vi "Read Credentials.vi"(8 "error in (no error)":errorcluster, 11 "AWS Core in":refnum<class "Session.lvclass">) -> (0 "error out":errorcluster, 2 "Credentials":T1, 3 "AWS Core out":refnum<class "Session.lvclass">)   [LabVIEW 2015, in "NI_Azure_Core.lvlib" / "Session.lvclass"]
uses:
  Session.lvclass
  Azure Credentials.ctl
  Session.lvclass/Session.ctl
  NI_Azure_Core.lvlib
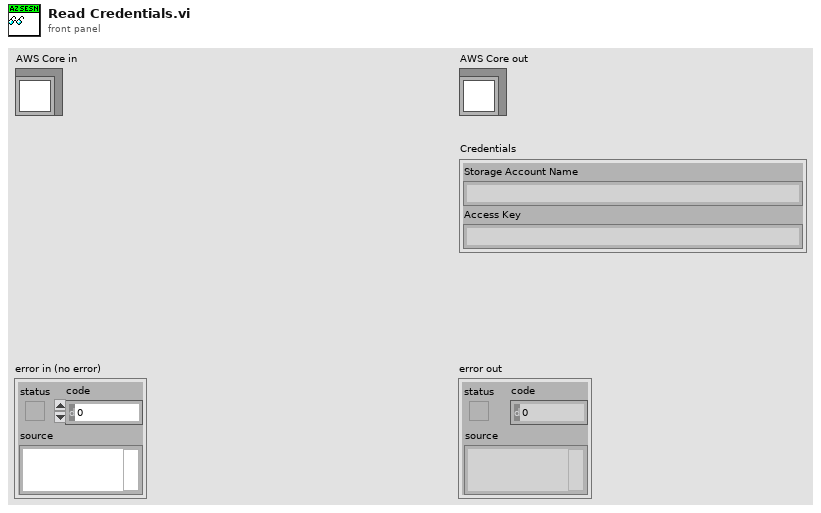
[diagram p1: front panel]
types:
  T1 = typedef "NI_Azure_Core.lvlib/Azure Credentials.ctl" = cluster{"Storage Account Name":string, "Access Key":string}
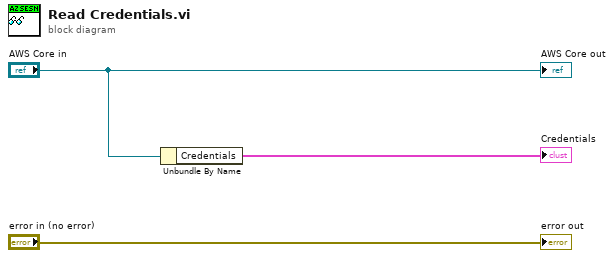
[diagram p0: block diagram]
diagram:
  n1 = Unbundle By Name("AWS Core in") -> ("Credentials"=→"Credentials":T1)
  "error out" <- "error in (no error)"
  "AWS Core out" <- "AWS Core in"
